vi "Vision Proc (SubVI).vi"(0 "Image In":T2, 2 "Hue in":i32(knob)=85 scale=0.0..255.0, 3 "Particle Count Limit":i32=10, 5 "Saturation in":i32=110, 6 "Value in":i32=45, 8 "Dilate_its":i32=1, 10 "Processing":enum32{"Color", "Monochrome"}(tab), 11 "Area Size Limit %":dbl=0.5, 12 "Score Limits":T1={"Rect Coverage"=60.0, "X Edge Strength"=40.0, "Y Edge Strength"=60.0, "Center"=75.0, "Outer"=75.0}, 13 "Margins":cluster{"Hue":i32, "Sat":i32, "Val":i32}={"Hue"=33, "Sat"=53, "Val"=9} {"Sat" scale=0.0..80.0; "Val" scale=0.0..80.0; "Hue" scale=0.0..80.0}, 14 "Erode_its":i32=1, 16 "Camera Type":enum16{"206", "1011"}(ring)=enum."1011", 17 "Annotate":bool=TRUE) -> (20 "Processed Image":T2(plugin-control), 22 "Target Info":T3(array[cluster]), 23 "Value out":cluster{i32, i32}, 25 "Saturation out":cluster{i32, i32}, 26 "Hue":cluster{i32, i32})   [LabVIEW 2012]
uses:
  <vilib>/vision/NI_Vision_Development_Module.lvlib
  <vilib>/vision/Image Controls.llb/IMAQ Image.ctl
panel:
  in  "Vert Limits":T1={"Rect Coverage"=60.0, "X Edge Strength"=40.0, "Y Edge Strength"=60.0, "Center"=75.0, "Outer"=75.0}
  in  "File List":i32(listbox)
  in  "Directory":path
  # "Lower/Upper"
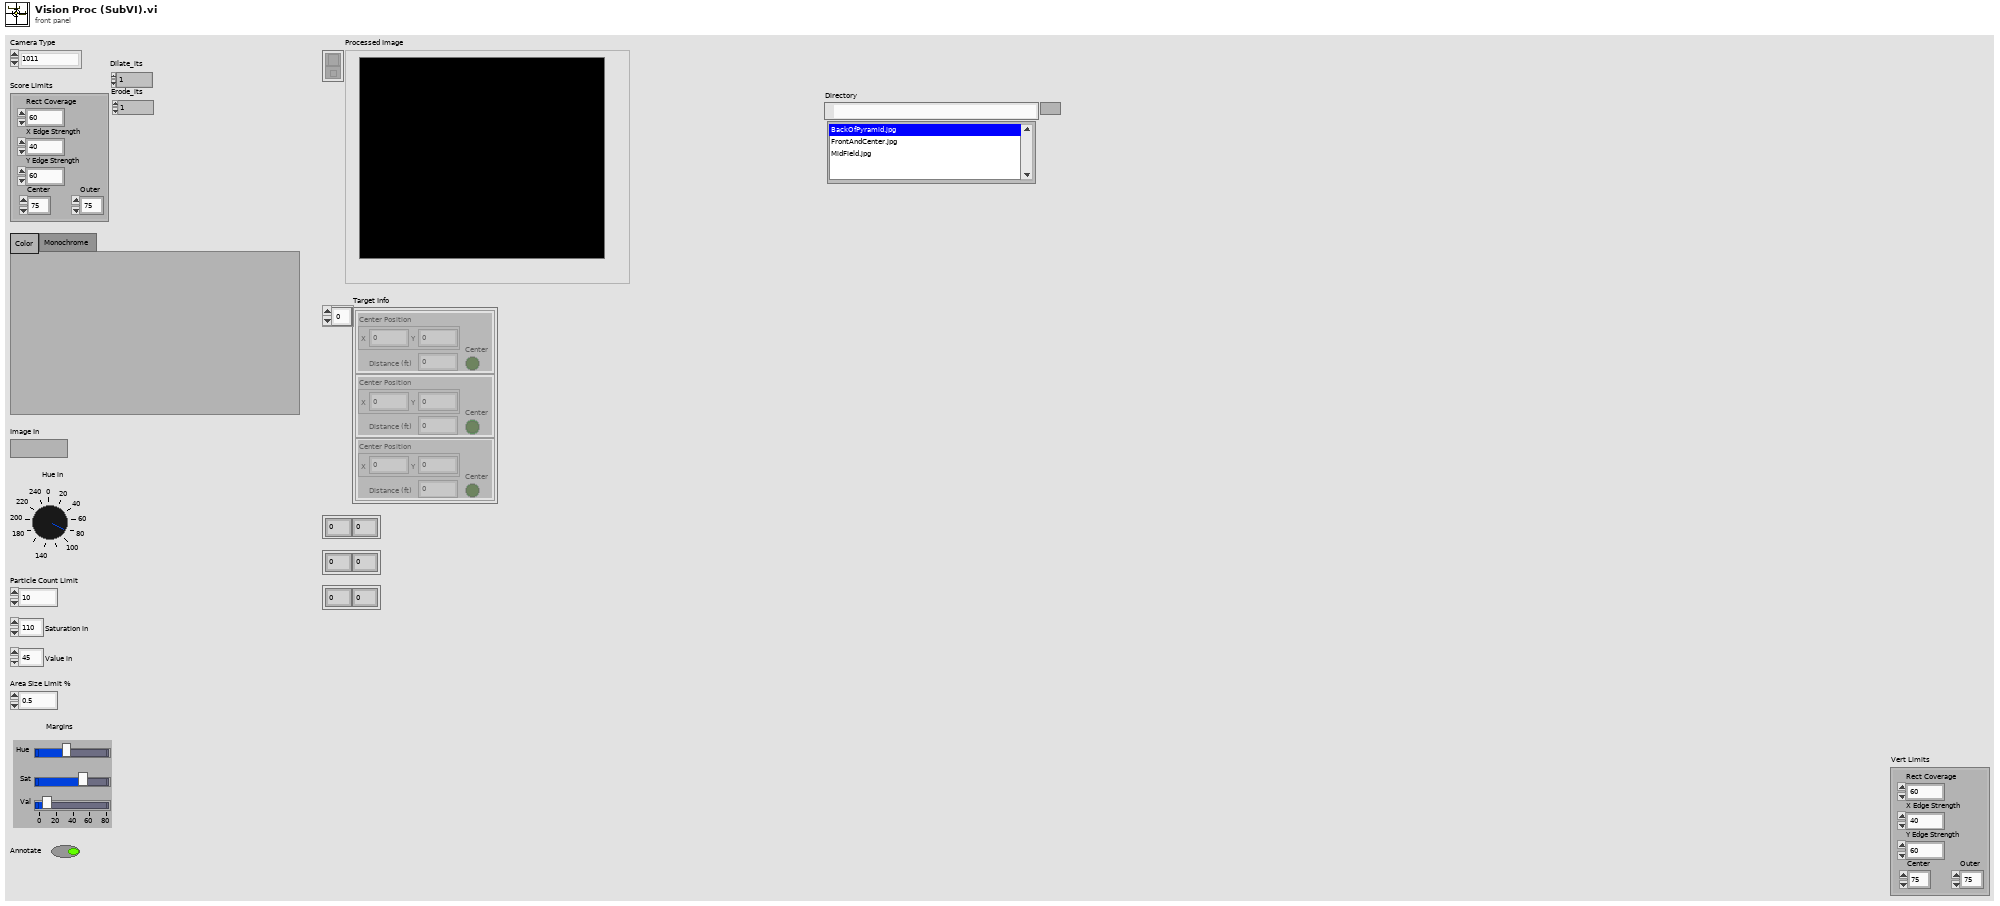
[diagram p1: front panel]
types:
  T1 = cluster{"Rect Coverage":dbl, "X Edge Strength":dbl, "Y Edge Strength":dbl, "Center":dbl, "Outer":dbl}
  T2 = typedef "IMAQ Image.ctl" = refnum<image>
  T3 = cluster{"Center Position":cluster{"X":dbl, "Y":dbl}, "Distance (ft)":dbl, "Center":bool}[]
  T4 = typedef "Image Type" = u32
  T5 = enum32{"AutoM", "Close", "Dilate", "Erode", "Gradient", "Gradient out", "Gradient in", "Hit miss", "Open", "PClose", "POpen", "Thick", "Thin"}
  T6 = cluster{"Position":cluster{"X":dbl, "Y":dbl}, "Distance (ft)":dbl, bool}[]
  T7 = cluster{cluster{"Left":dbl, "Top":dbl, "Right":dbl, "Bottom":dbl}, "Scores":dbl[], cluster{"Long":dbl, "Short":dbl}}[]
  T8 = cluster{"Target Center (-1 to 1)":cluster{"X":dbl, "Y":dbl}, "Distance (ft)":dbl, "Center Target":bool}
  T9 = cluster{"Target Center (-1 to 1)":cluster{"X":dbl, "Y":dbl}, "Distance (ft)":dbl, "Center Target":bool}[]
  T10 = cluster{"Left":dbl, "Top":dbl, "Right":dbl, "Bottom":dbl}
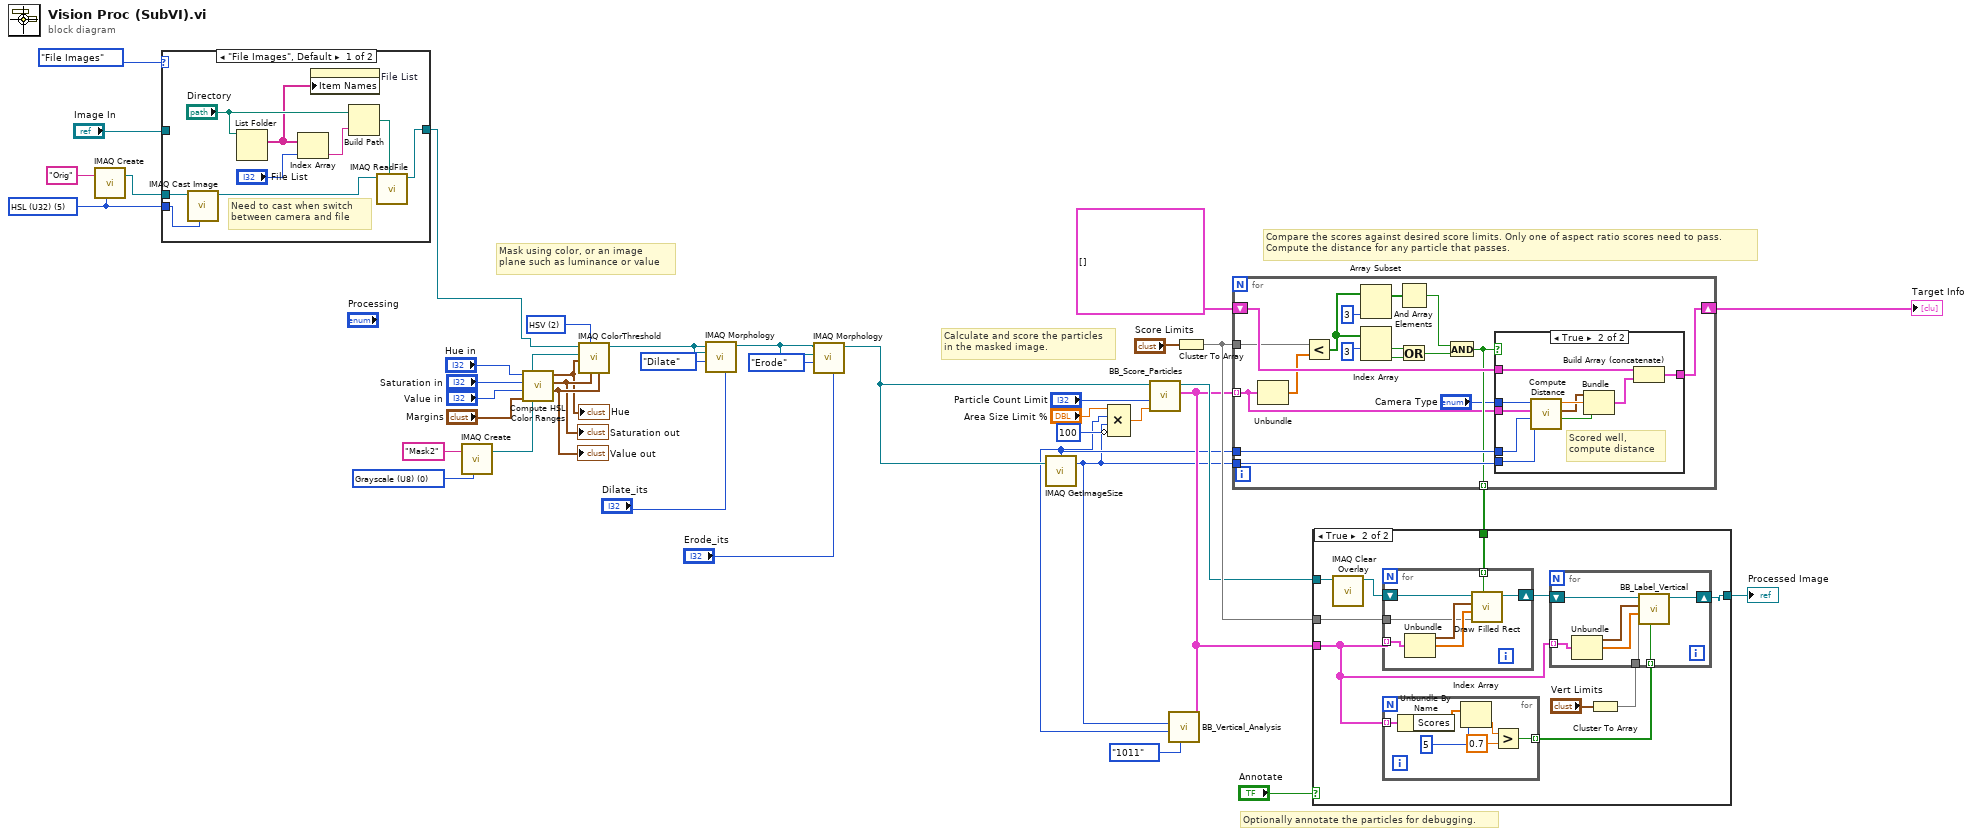
[diagram p0: block diagram]
diagram:
  w9 = T4 5 items=["Grayscale (U8)", "Grayscale (I16)", "Grayscale (SGL)", "Complex (CSG)", "RGB (U32)", "HSL (U32)", "RGB (U64)", "Grayscale (U16)"] ("Image Type")
  w39 = T4 0 items=["Grayscale (U8)", "Grayscale (I16)", "Grayscale (SGL)", "Complex (CSG)", "RGB (U32)", "HSL (U32)", "RGB (U64)", "Grayscale (U16)"] ("Image Type")
  w31 = u16 2 items=["RGB", "HSL", "HSV", "HSI"] ("Color Mode")
  # "Optionally annotate the particles for debugging."
  # "Compare the scores against desired score limits. Only one of aspect ratio scores need to pass.\nCompute the distance for any particle that passes."
  # "Calculate and score the particles\nin the masked image."
  # "Mask using color, or an image\nplane such as luminance or value"
  n1 = call "IMAQ Create"("Image Name"="Orig", "Image Type"=w9) -> ("New Image"=w8:T2)  [unwired: 2 in, 2 out]
  n2 = case shown="\"File Images\", Default" enum32{"File Images", "Live Camera"}."File Images" ("Image Source") {
    tunnel: [w43 w50] -> w7
    tunnel: "Image In" -> [_ w50]
    tunnel: w9 -> [w42 _]
    tunnel: w8 -> [w41 _]
    frame "File Images", Default {
      # "Need to cast when switch\nbetween camera and file"
      n3 = call "IMAQ Cast Image"("Image Type"=w42, "Image Src"=w41) -> ("Image Dst Out"=w44:T2)  [unwired: 8 in, 1 out]
      n4 = List Folder(path="Directory") -> (filenames=w45:string[])  [unwired: 3 in, 3 out]
      n5 = Index Array(array=w45, index="File List") -> (element=w48:string)
      n6 = property on="File List" class="LstBox (strict)"("Item Names"=w45) -> ()  [unwired: 2 in, 2 out]
      n7 = Build Path(base path="Directory", name or relative path=w48) -> (appended path=w47:path)
      n8 = call "IMAQ ReadFile"("File Path"=w47, "Image"=w44) -> ("Image Out"=w43:T2)  [unwired: 5 in, 4 out]
    }
    frame "Live Camera" {
    }
  }
  n9 = call "IMAQ Create"("Image Name"="Mask2", "Image Type"=w39) -> ("New Image"=w18:T2)  [unwired: 2 in, 2 out]
  n10 = call "Compute HSL Color Ranges.vi"("Margins"="Margins", "Luminance"="Value in", "Saturation"="Saturation in", "Hue"="Hue in") -> ("Lum Range"=w38:cluster{i32, i32}, "Sat Range"=w37:cluster{i32, i32}, "Hue Range"=w32:cluster{i32, i32})  [unwired: 5 in]
  "Hue" <- w32
  "Saturation out" <- w37
  "Value out" <- w38
  n11 = call "IMAQ ColorThreshold"("Blue or Luma or Val or Inten Range"=w38, "Green or Sat Range"=w37, "Color Mode"=w31, "Red or Hue Range"=w32, "Image Dst"=w18, "Image Src"=w7) -> ("Image Dst Out"=w17:T2)  [unwired: 4 in, 1 out]
  n12 = call "IMAQ Morphology"("Number of iterations (1)"="Dilate_its", "Operation"=T5."Dilate", "Image Dst"=w17, "Image Src"=w17) -> ("Image Dst Out"=w14:T2)  [unwired: 6 in, 1 out]
  n13 = call "IMAQ Morphology"("Number of iterations (1)"="Erode_its", "Operation"=T5."Erode", "Image Dst"=w14, "Image Src"=w14) -> ("Image Dst Out"=w5:T2)  [unwired: 6 in, 1 out]
  n14 = call "IMAQ GetImageSize"("Image"=w5) -> ("Y Resolution"=w2:i32, "X Resolution"=w3:i32)  [unwired: 3 in, 1 out]
  n15 = Compound Arithmetic op=MULTIPLY("Area Size Limit %", w3, w2, invert 100 ("value")) -> (w29:dbl)
  n16 = call "BB_Score_Particles.vi"("Area Size Limit"=w29, "Particle Count Limit"="Particle Count Limit", "Image Refnum in"=w5) -> ("Scored Particle Info"=w4:T7, "Image Refnum out"=w20:T2)  [unwired: 7 in]
  n17 = call "BB_Vertical_Analysis.vi"("Scored Particle Info"=w4, "Camera Type"=enum16{"206", "1011"}."1011", "X Resolution"=w3, "Y Resolution"=w2) -> ()  [unwired: 8 in]
  n18 = Cluster To Array(cluster="Score Limits") -> (array=w26:dbl[])
  n19 = for {
    shift-right: [w66] -> w19
    shift-left: T6 [] -> [w67]
    tunnel: w3 -> [w65]
    tunnel: w4 -> [w51] mode=indexing
    tunnel: w26 -> [w63]
    tunnel: w2 -> [w62]
    tunnel: [w53] -> w27 mode=indexing
    n20 = Unbundle(w51) -> ("Scores"=w64:dbl[])  [unwired: 2 out]
    n21 = Less?(x=w63, y=w64) -> (x < y?=w59:bool[])
    n22 = Array Subset(array=w59, length=3) -> (w60:bool[])  [unwired: 1 in]
    n23 = Index Array(array=w59, index #1=3 ("length")) -> (element #1=w57:bool, element #2=w56:bool)  [unwired: 1 in]
    n24 = And Array Elements(Boolean array=w60) -> (logical AND=w54:bool)
    n25 = Or(x=w57, y=w56) -> (x .or. y?=w55:bool)
    n26 = And(x=w54, y=w55) -> (x .and. y?=w53:bool)
    n27 = case shown="True" w53 {
      tunnel: w67 -> [w68 w78]
      tunnel: [w68 w77] -> w66
      tunnel: w65 -> [_ w75]
      tunnel: "Camera Type" -> [_ w73]
      tunnel: w62 -> [_ w71]
      tunnel: w51 -> [_ w70]
      frame False {
        # "Didn't score well enough"
      }
      frame True {
        # "Scored well,\ncompute distance"
        n28 = call "Compute Distance.vi"("Y Image Resolution"=w71, "X Image Resolution"=w75, "Particle Scores"=w70, "Camera Type"=w73) -> ("Center Target"=w69:bool, "Target Center (-1 to 1)"=w72:cluster{"X":dbl, "Y":dbl}, "Distance (ft)"=w74:dbl)  [unwired: 5 in]
        n29 = Bundle("Target Center (-1 to 1)"=w72, "Distance (ft)"=w74, "Center Target"=w69) -> (w76:T8)  [unwired: 1 in]
        n30 = Build Array (concatenate)(w78, w76) -> (w77:T9)
      }
    }
  }
  "Target Info" <- w19
  n31 = case shown="True" "Annotate" {
    tunnel: w20 -> [w79 w89]
    tunnel: [w79 w85] -> w22
    tunnel: w4 -> [_ w83]
    tunnel: w26 -> [_ w87]
    tunnel: w27 -> [_ w86]
    frame False {
    }
    frame True {
      n32 = call "IMAQ Clear Overlay"("Image"=w89) -> ("Image Out"=w88:T2)  [unwired: 2 in, 8 out]
      n33 = for {
        shift-right: [w108] -> w84
        shift-left: w88 -> [w109]
        tunnel: w83 -> [w105] mode=indexing
        tunnel: w87 -> [w104]
        tunnel: w86 -> [w103] mode=indexing
        n34 = Unbundle(w105) -> (w106:T10, "Scores"=w107:dbl[])  [unwired: 1 out]
        n35 = call "Draw Filled Rect.vi"("Limit Passed"=w103, "Limits"=w104, "Scores"=w107, "Bounding Box"=w106, "image in"=w109) -> ("image out"=w108:T2)  [unwired: 6 in]
      }
      n36 = for {
        tunnel: [w102] -> w80 mode=indexing
        tunnel: w83 -> [w100] mode=indexing
        n37 = Unbundle By Name(w100) -> ("Scores"=w99:dbl[])
        n38 = Index Array(array=w99, index=5) -> (element=w98:dbl)
        n39 = Greater?(x=w98, y=0.7) -> (0:w102:bool)
      }
      n40 = Cluster To Array(cluster="Vert Limits") -> (array=w81:dbl[])
      n41 = for {
        shift-right: [w91] -> w85
        shift-left: w84 -> [w96]
        tunnel: w83 -> [w93] mode=indexing
        tunnel: w81 -> [w92]
        tunnel: w80 -> [w90] mode=indexing
        n42 = Unbundle(w93) -> (w94:T10, "Scores"=w95:dbl[])  [unwired: 1 out]
        n43 = call "BB_Label_Vertical.vi"("Limit Passed"=w90, "Limits"=w92, "Scores"=w95, "Bounding Box"=w94, "image in"=w96) -> ("image out"=w91:T2)  [unwired: 6 in]
      }
    }
  }
  "Processed Image" <- w22
